vi "WPI_SimpleGyro_RefNum Registry Set.vi"(8 "error in (no error)":errorcluster, 10 "refnum name":string="SimpleGyroRefNum", 11 "SimpleGyroDevRef":T1) -> (0 "error out":errorcluster, 3 "SimpleGyroDevRef":T1)   [LabVIEW 2015, in "SimpleGyro.lvlib"]
doc: "Sets a reference into a registry so that other VIs can call the reference. After you set a reference, you can call that reference with SimpleGyro_RefNum Registry Get VI."
uses:
  SimpleGyro.lvlib
  WPI_SimpleGyroDevRef.ctl
  <vilib>/Rock Robotics/SystemInterfaces/spilib/spi_bus.ctl
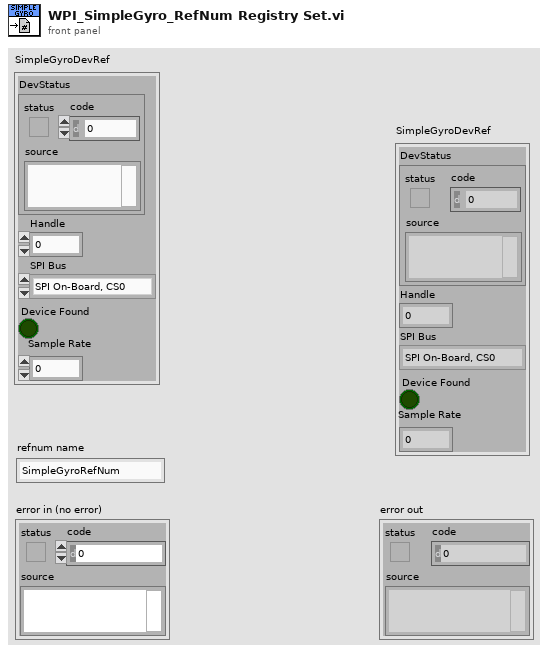
[diagram p1: front panel]
types:
  T1 = typedef "SimpleGyro.lvlib/WPI_SimpleGyroDevRef.ctl" = cluster{"DevStatus":errorcluster, "Handle":i32, "SPI Bus":T2, "Device Found":bool, "Sample Rate":dbl}
  T2 = typedef "spi_bus.ctl" = enum16{"SPI On-Board, CS0", "SPI On-Board, CS1", "SPI On-Board, CS2", "SPI On-Board, CS3", "SPI MXP", "Invalid"}
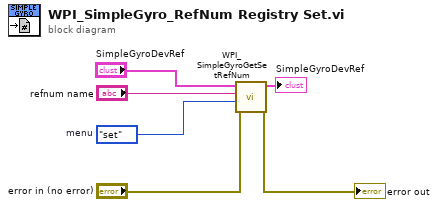
[diagram p0: block diagram]
diagram:
  w4 = enum16{"set", "get", "delete"}."set"  # menu
  n1 = call "WPI_SimpleGyroGetSetRefNum.vi"("error in (no error)"="error in (no error)", "menu"=w4, "refnum name"="refnum name", "SimpleGyroDevRef"="SimpleGyroDevRef") -> ("error out"=→"error out":errorcluster, "SimpleGyroDevRef"=→"SimpleGyroDevRef":T1)  [unwired: 6 in]
